vi "SetRelativePositionUm.vi"(8 "error in (no error)":errorcluster, 9 "RelativeMoveum":dbl min=0.0 max=200.0, 10 "Stage Label":string, 11 "Stage_MadCityLab in":refnum<class "Stage_MadCityLab.lvclass">) -> (0 "error out":errorcluster, 3 "Stage_MadCityLab out":refnum<class "Stage_MadCityLab.lvclass">)   [LabVIEW 2020, in "Stage_MadCityLab.lvlib" / "Stage_MadCityLab.lvclass"]
uses:
  Stage_MadCityLab.lvclass
  Dependency/Madlib.dll
  <vilib>/ActorFramework/Actor/Actor.lvclass
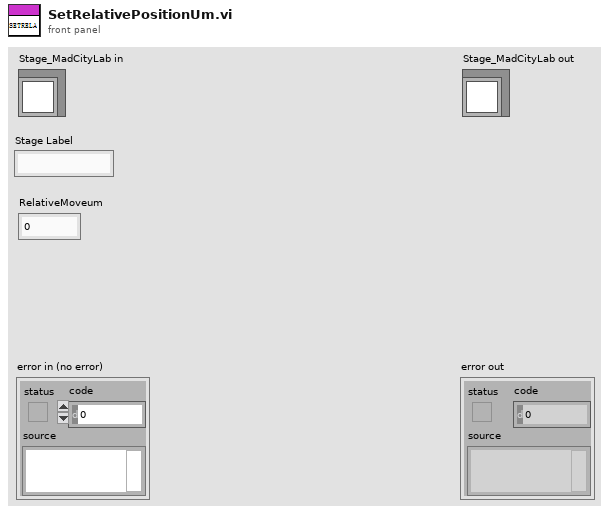
[diagram p1: front panel]
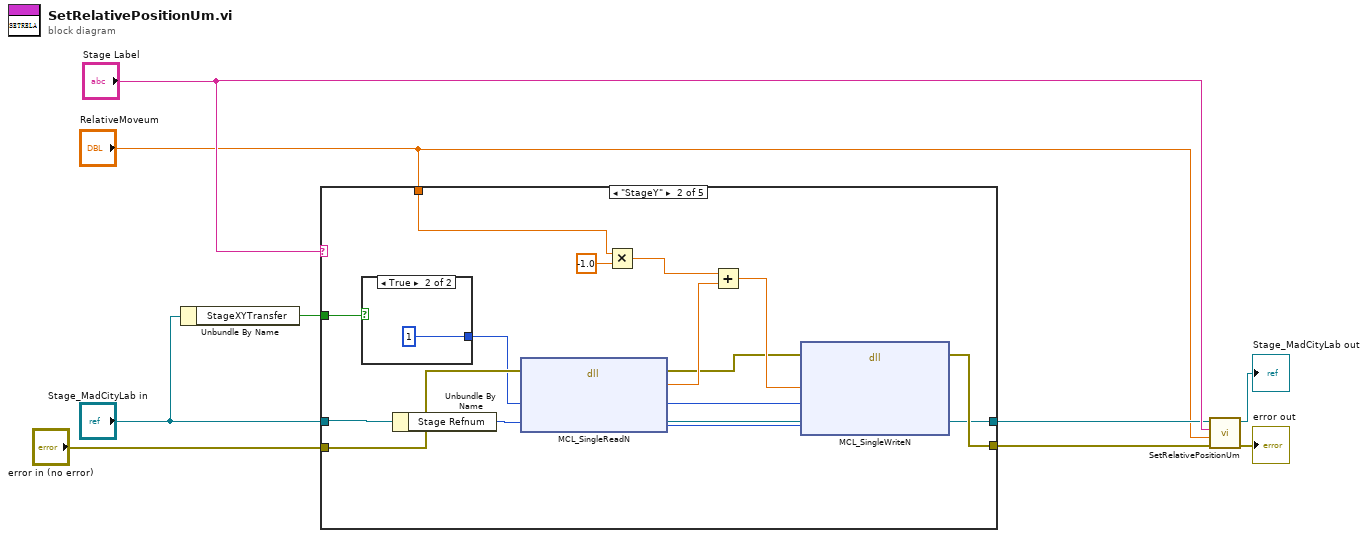
[diagram p0: block diagram]
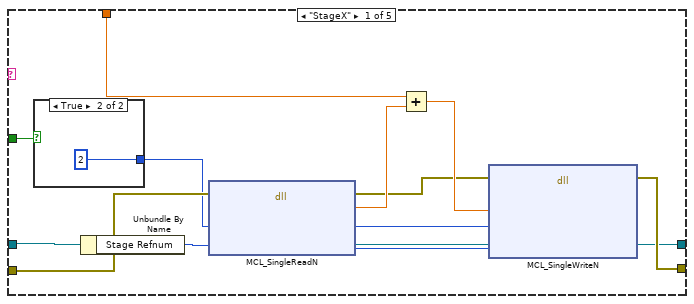
[diagram p2: hidden frame]
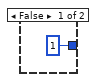
[diagram p3: hidden frame]
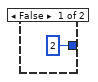
[diagram p4: hidden frame]
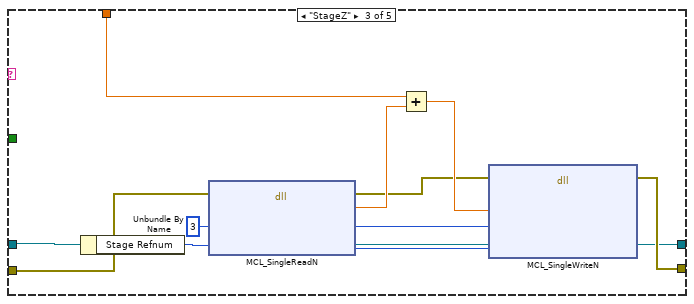
[diagram p5: hidden frame]
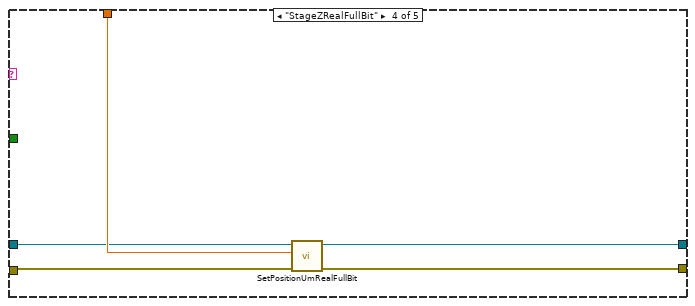
[diagram p6: hidden frame]
diagram:
  n1 = Unbundle By Name("Stage_MadCityLab in") -> ("StageXYTransfer"=w1:bool)
  n2 = case shown="\"StageY\"" "Stage Label" {
    tunnel: "Stage_MadCityLab in" -> [w12 w29 w40 w54 w57]
    tunnel: [w12 w29 w40 w53 w57] -> w6
    tunnel: "RelativeMoveum" -> [w15 w26 w44 w55 _]
    tunnel: "error in (no error)" -> [w14 w31 w43 w52 w56]
    tunnel: [w13 w30 w42 w51 w56] -> w4
    tunnel: w1 -> [w11 w28 _ _ _]
    frame "StageX" {
      n3 = case shown="True" w11 {
        tunnel: [u32 1 ("axis") u32 2 ("axis")] -> w10
        frame False {
        }
        frame True {
        }
      }
      n4 = Unbundle By Name(w12) -> ("Stage Refnum"=w16:i32)
      n5 = dll-call lib="E:/Development/DevHardSoftware/MicroscopyFramework/Model/Hardware Layer/Real Hardware/Stage_MadCityLab/Stage_MadCityLab/Dependency/Madlib.dll" fn="MCL_SingleReadN"(error in=w14, "axis"=w10, "handle"=w16) -> (error out=w17:errorcluster, "return type"=w19:dbl, "axis"=w20:u32, "handle"=w21:i32)  [unwired: 2 in, 1 out]
      n6 = Add(x=w15, y=w19) -> (x+y=w18:dbl)
      n7 = dll-call lib="E:/Development/DevHardSoftware/MicroscopyFramework/Model/Hardware Layer/Real Hardware/Stage_MadCityLab/Stage_MadCityLab/Dependency/Madlib.dll" fn="MCL_SingleWriteN"(error in=w17, "position"=w18, "axis"=w20, "handle"=w21) -> (error out=w13:errorcluster)  [unwired: 6 in, 1 out]
    }
    frame "StageY" {
      n8 = case shown="True" w28 {
        tunnel: [u32 2 ("axis") u32 1 ("axis")] -> w27
        frame False {
        }
        frame True {
        }
      }
      n9 = Unbundle By Name(w29) -> ("Stage Refnum"=w32:i32)
      n10 = dll-call lib="E:/Development/DevHardSoftware/MicroscopyFramework/Model/Hardware Layer/Real Hardware/Stage_MadCityLab/Stage_MadCityLab/Dependency/Madlib.dll" fn="MCL_SingleReadN"(error in=w31, "axis"=w27, "handle"=w32) -> (error out=w33:errorcluster, "return type"=w35:dbl, "axis"=w36:u32, "handle"=w37:i32)  [unwired: 2 in, 1 out]
      n11 = Multiply(x=w26, y=-1.0) -> (x*y=w25:dbl)
      n12 = Add(x=w25, y=w35) -> (x+y=w34:dbl)
      n13 = dll-call lib="E:/Development/DevHardSoftware/MicroscopyFramework/Model/Hardware Layer/Real Hardware/Stage_MadCityLab/Stage_MadCityLab/Dependency/Madlib.dll" fn="MCL_SingleWriteN"(error in=w33, "position"=w34, "axis"=w36, "handle"=w37) -> (error out=w30:errorcluster)  [unwired: 6 in, 1 out]
    }
    frame "StageZ" {
      n14 = Unbundle By Name(w40) -> ("Stage Refnum"=w45:i32)
      n15 = dll-call lib="E:/Development/DevHardSoftware/MicroscopyFramework/Model/Hardware Layer/Real Hardware/Stage_MadCityLab/Stage_MadCityLab/Dependency/Madlib.dll" fn="MCL_SingleReadN"(error in=w43, "axis"=u32 3, "handle"=w45) -> (error out=w46:errorcluster, "return type"=w48:dbl, "axis"=w49:u32, "handle"=w50:i32)  [unwired: 2 in, 1 out]
      n16 = Add(x=w44, y=w48) -> (x+y=w47:dbl)
      n17 = dll-call lib="E:/Development/DevHardSoftware/MicroscopyFramework/Model/Hardware Layer/Real Hardware/Stage_MadCityLab/Stage_MadCityLab/Dependency/Madlib.dll" fn="MCL_SingleWriteN"(error in=w46, "position"=w47, "axis"=w49, "handle"=w50) -> (error out=w42:errorcluster)  [unwired: 6 in, 1 out]
    }
    frame "StageZRealFullBit" {
      n18 = call-dynamic "SetPositionUmRealFullBit.vi"("error in (no error)"=w52, "relative Z"=w55, "Stage_MadCityLab in"=w54) -> ("error out"=w51:errorcluster, "Stage_MadCityLab out"=w53:refnum<class "Stage_MadCityLab.lvclass">)  [unwired: 7 in]
    }
    frame Default {
    }
  }
  n19 = call-parent "SetRelativePositionUm.vi"("error in (no error)"=w4, "RelativeMoveum"="RelativeMoveum", "Stage Label"="Stage Label", "Stage in"=w6) -> ("error out"=→"error out":errorcluster, "Stage out"=→"Stage_MadCityLab out":refnum<class "Stage_MadCityLab.lvclass">)  [unwired: 6 in]
